vi "仪器控制2.vi"() -> ()   [LabVIEW 2012]
uses:
  <vilib>/Instr/_visa.llb/VISA Configure Serial Port (Instr).vi
panel:
  out "已循环周期数":i32
  out "电流下限":dbl
  out "电流上限":dbl
  in  "截取下限时间 2":dbl=50.0
  in  "截取上限时间 2":dbl=59.5
  in  "偏差范围下限 2":dbl=20.0
  in  "偏差范围上限 2":dbl=20.0
  in  "截取下限时间":dbl=0.75
  in  "截取上限时间":dbl=49.0
  out "当前时间值":dbl
  out "电流超出范围":bool=TRUE
  out "原始数据":dbl
  out "大小":i32
  in  "终止程序":bool
  out "x-y":u32
  out "波形图":dbl[](graph)
  out "子字符串之前 2":string
  out "双精度浮点数":dbl
  out "*(类型 *) &x":dbl
  out "实际输出电流":dbl
  out "匹配后偏移量":i32
  out "子字符串之后":string
  out "匹配子字符串":string
  out "子字符串之前":string
  out "读取缓冲区":string
  out "Serial Settings:Number of Bytes at Serial Port":u32
  out "停止按钮指示灯":bool
  out "运行按钮指示灯":bool
  in  "停止运行":bool
  in  "运行程序":bool
  in  "第一段波形持续时间(s)":dbl=49.25
  in  "循环周期数":i32=30000
  in  "0安培电流保持时长":dbl=60.0
  in  "前三段波形持续时间（s）":dbl=60.0
  in  "前两段波形持续时间（s）":dbl=59.5
  in  "Time Resolution(s)":dbl=0.03
  in  "IR":dbl=50.0
  out "第一周期近似波形图":dbl[](graph)
  # "配置"
  # "检测"
  # "Time Resolution(s)不能小于0.03否则时间将特别不准"
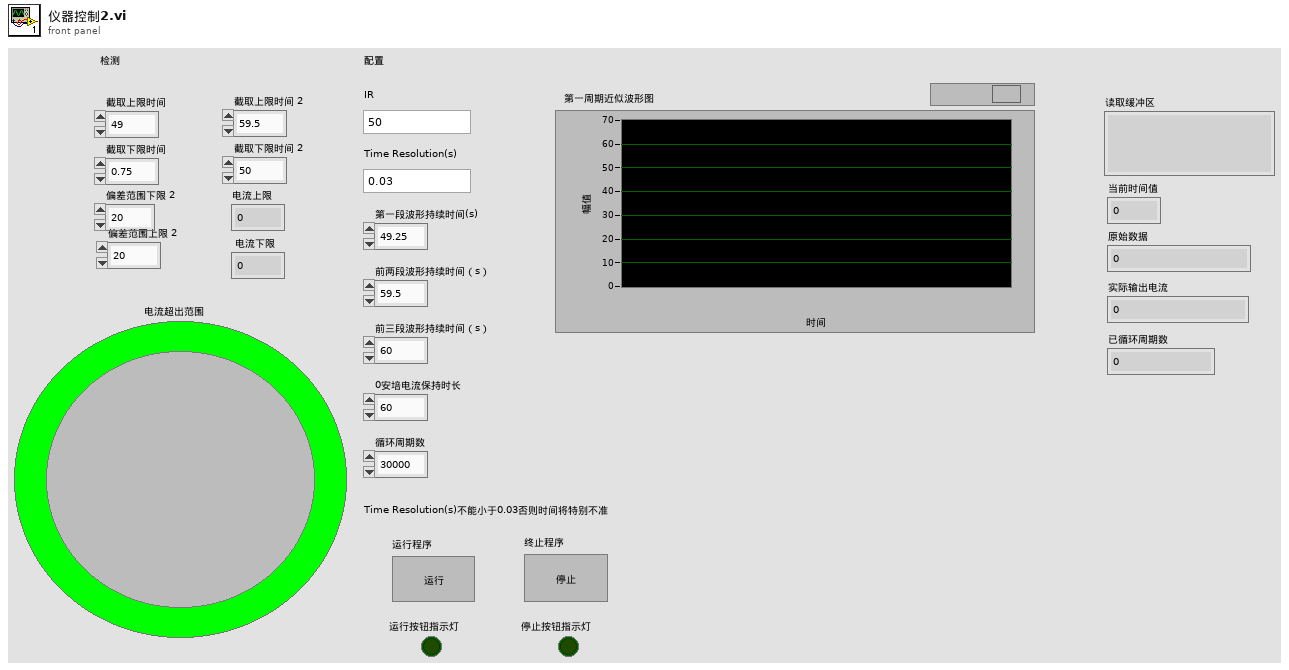
[diagram p1: front panel]
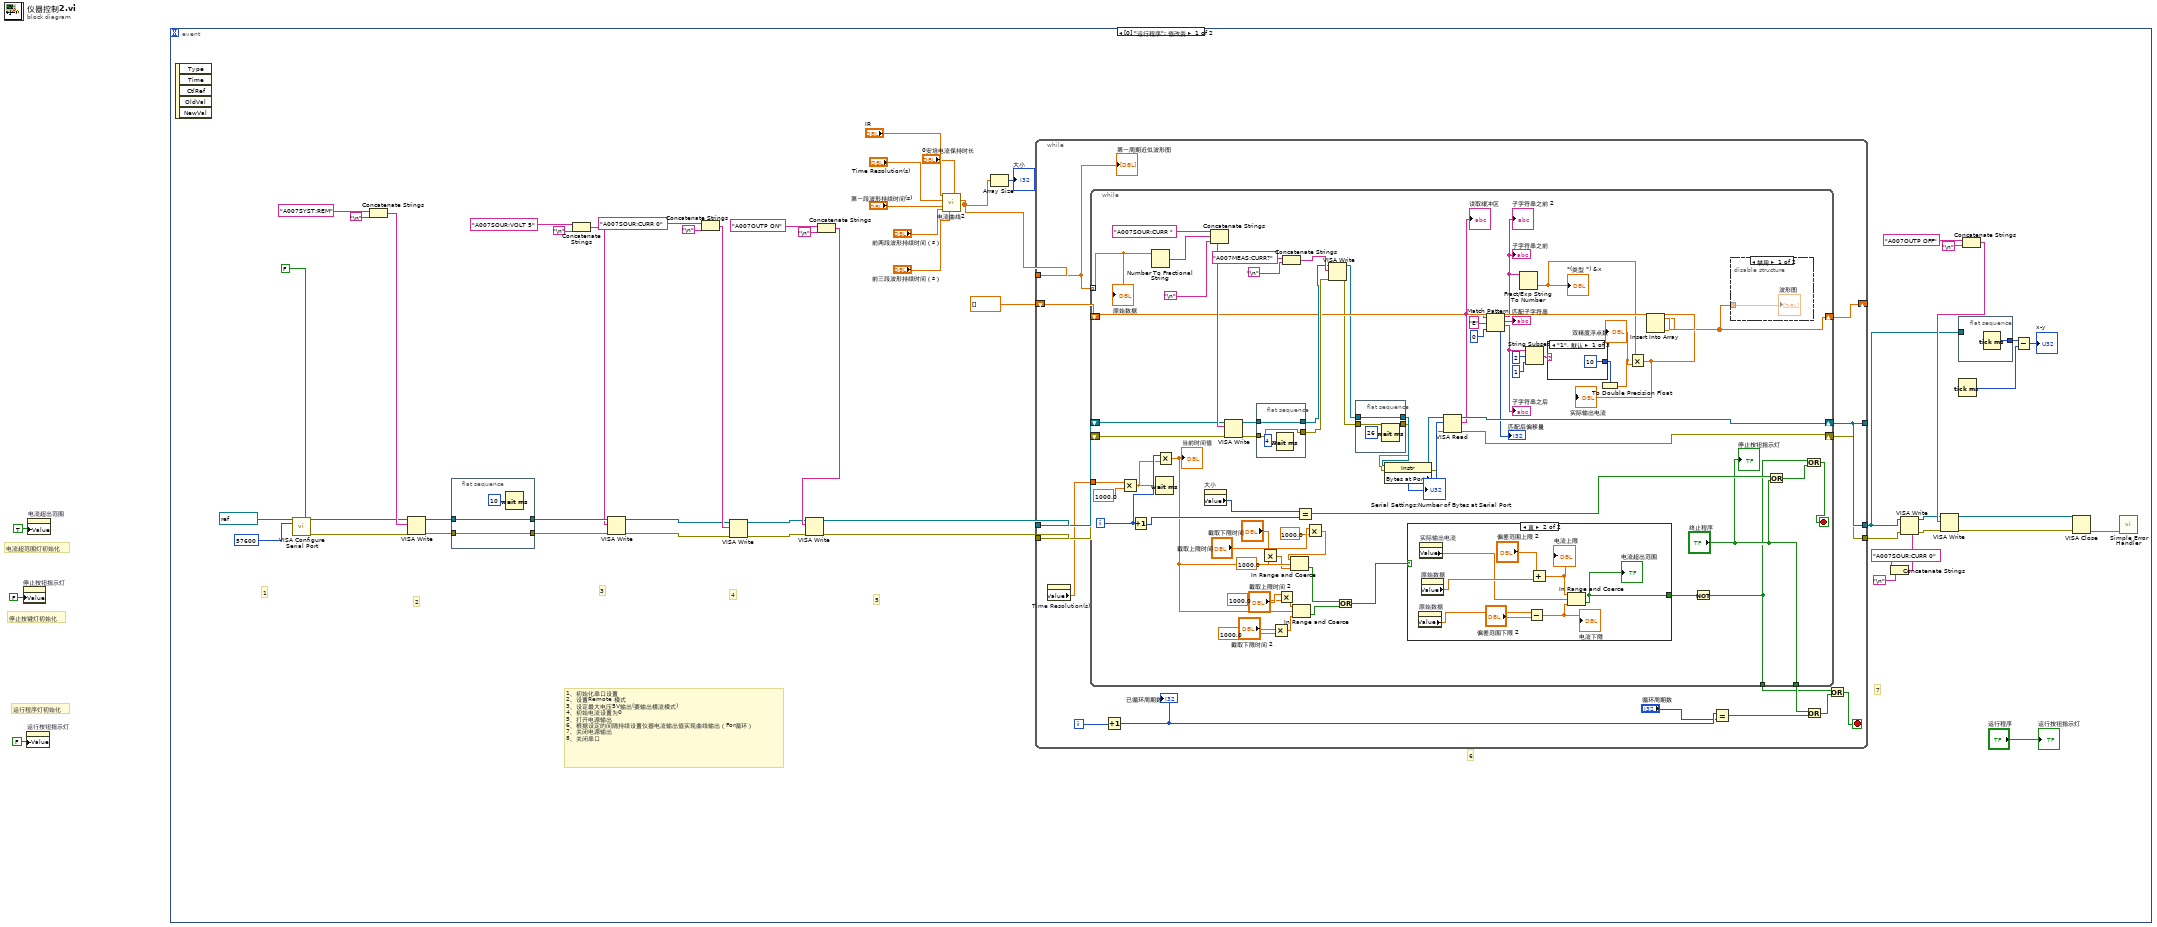
[diagram p0: block diagram]
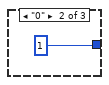
[diagram p2: hidden frame]
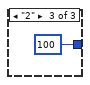
[diagram p3: hidden frame]
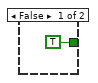
[diagram p5: hidden frame]
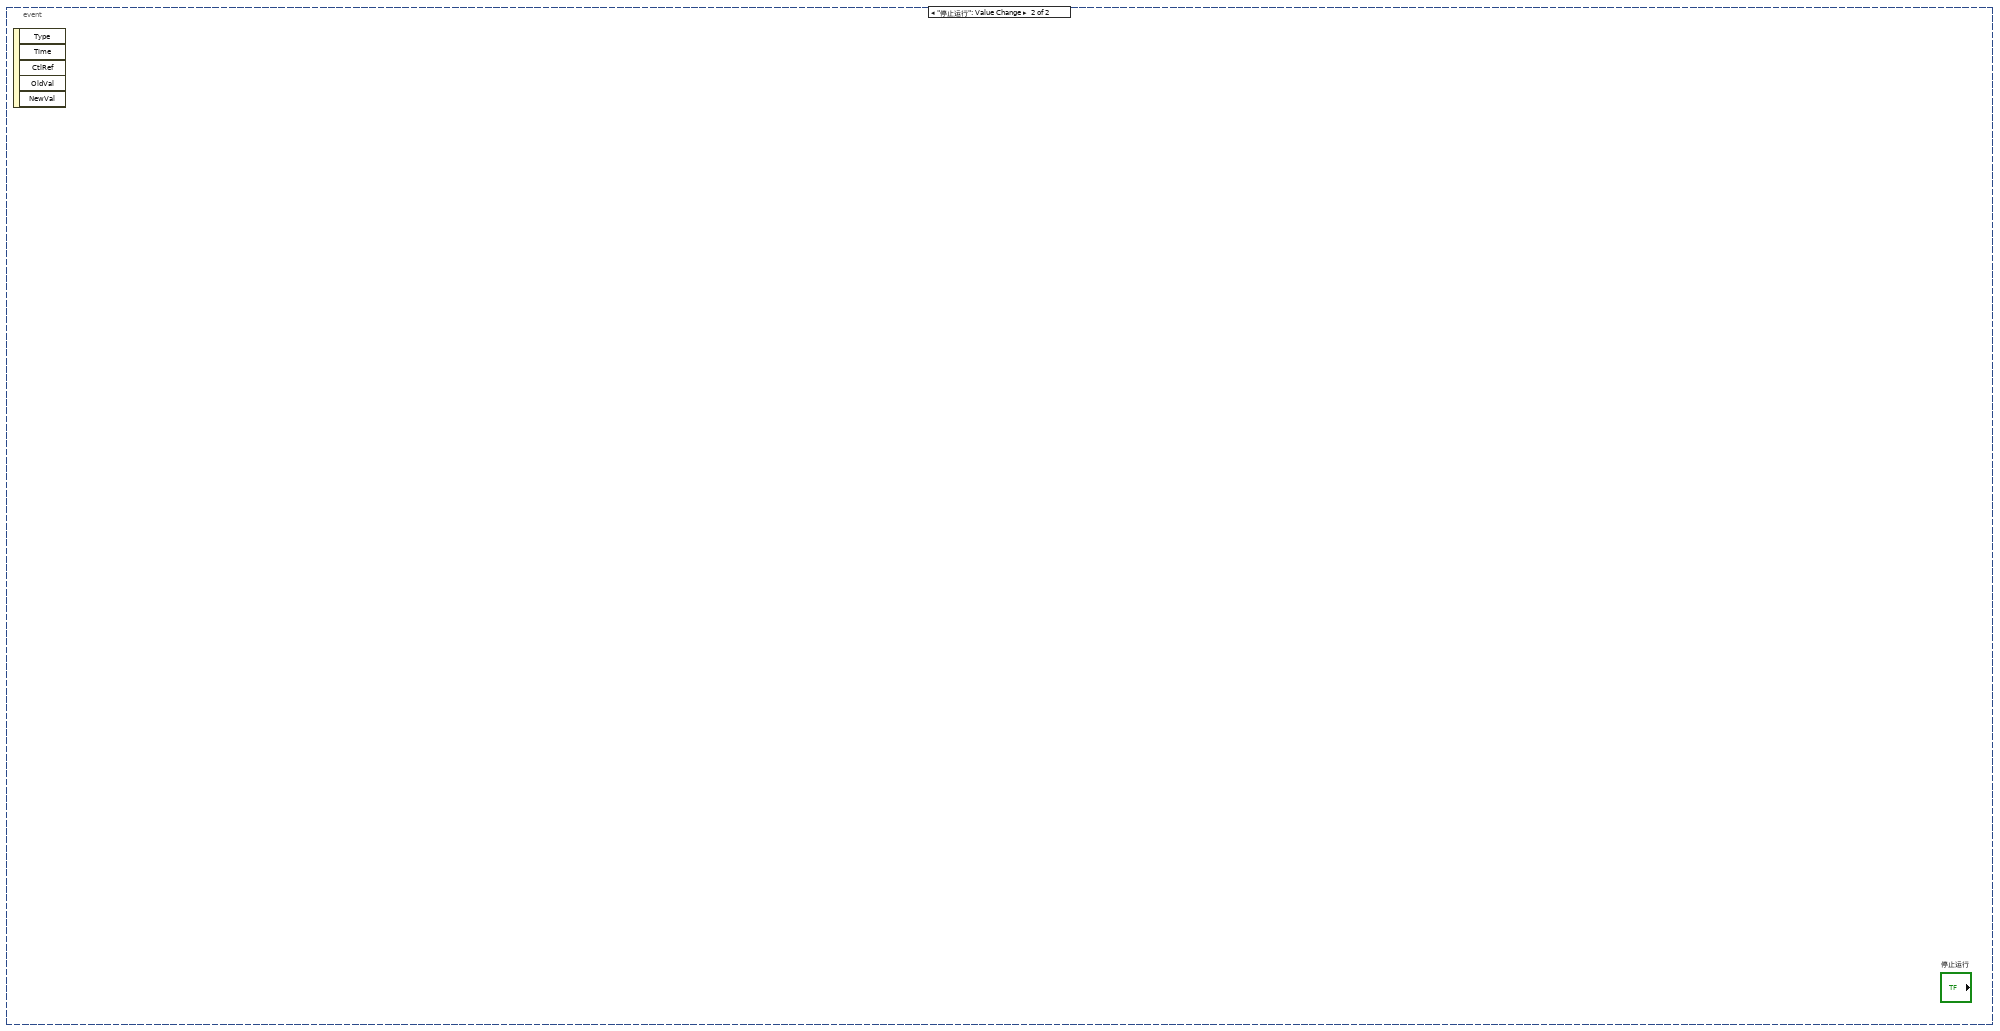
[diagram p6: hidden frame]
diagram:
  # "电流超范围灯初始化"
  # "停止按键灯初始化"
  # "运行程序灯初始化"
  n1 = property on="停止按钮指示灯" class="Bool (严格)"("Value"=FALSE ("停止按钮指示灯")) -> ()  [unwired: 2 in, 2 out]
  n2 = property on="运行按钮指示灯" class="Bool (严格)"("Value"=FALSE ("运行按钮指示灯")) -> ()  [unwired: 2 in, 2 out]
  n3 = property on="电流超出范围" class="Bool (严格)"("Value"=TRUE ("电流超出范围")) -> ()  [unwired: 2 in, 2 out]
  n4 = event shown="[0] \"运行程序\": 值改变" {
    selector: _ -> [_ _]
    dyn-events: _ -> [_ _]
    timeout: _ -> [_ _]
    event "运行程序": Value Change {
      # "6"
      # "7"
      # "5"
      # "4"
      # "3"
      # "2"
      # "1"
      # "1、初始化串口设置\n2、设置Remote 模式\n3、设定最大电压5V输出(要输出横流模式)\n4、初始电流设置为0\n5、打开电源输出\n6、根据设定的间隔持续设置仪器电流输出值实现曲线输出（For循环）\n7、关闭电源输出\n8、关闭串口"
      n5 = event-data() -> ()  [unwired: 1 in, 5 out]
      n6 = call-poly "VISA Configure Serial Port"("VISA resource name"=refnum<visa-resource-name> "COM3", "Enable Termination\nChar (T)"=FALSE ("Enable Termination\nChar (T)"), "baud rate (9600)"=u32 57600) -> ("VISA resource name out"=w48:refnum<visa-resource-name>, "error out"=w47:errorcluster)  [unwired: 11 in]
      n7 = Concatenate Strings("A007SYST:REM" ("字符串"), "\n") -> (w53:string)
      n8 = VISA Write(VISA resource name=w48, write buffer=w53, error in (no error)=w47) -> (VISA resource name out=w56:refnum<visa-resource-name>, error out=w55:errorcluster)  [unwired: 1 out]
      n9 = flat-sequence {
        tunnel: w56 -> [w161]
        tunnel: [w161] -> w45
        tunnel: w55 -> [w160]
        tunnel: [w160] -> w44
        frame #0 {
          n10 = Wait (ms)(milliseconds to wait=u32 10 ("等待时间（毫秒）")) -> ()  [unwired: 1 out]
        }
      }
      n11 = Concatenate Strings("A007SOUR:VOLT 5" ("字符串"), "\n") -> (w41:string)
      n12 = VISA Write(VISA resource name=w45, write buffer=w41, error in (no error)=w44) -> (VISA resource name out=w37:refnum<visa-resource-name>, error out=w36:errorcluster)  [unwired: 1 out]
      n13 = Concatenate Strings("A007SOUR:CURR 0" ("字符串"), "\n") -> (w40:string)
      n14 = VISA Write(VISA resource name=w37, write buffer=w40, error in (no error)=w36) -> (VISA resource name out=w32:refnum<visa-resource-name>, error out=w31:errorcluster)  [unwired: 1 out]
      n15 = Concatenate Strings("A007OUTP ON" ("字符串"), "\n") -> (w33:string)
      n16 = VISA Write(VISA resource name=w32, write buffer=w33, error in (no error)=w31) -> (VISA resource name out=w30:refnum<visa-resource-name>, error out=w29:errorcluster)  [unwired: 1 out]
      n17 = call "电流曲线2.vi"("0安培电流保持时长"="0安培电流保持时长", "总持续时间3"="前三段波形持续时间（s）", "总持续时间2"="前两段波形持续时间（s）", "总持续时间1"="第一段波形持续时间(s)", "时间分辨率"="Time Resolution(s)", "IR"="IR") -> ("最终电流值"=w12:dbl[])  [unwired: 5 in]
      n18 = Array Size(array=w12) -> (size(s)=→"大小":i32)
      n19 = while {
        tunnel: w30 -> [w72]
        tunnel: w29 -> [w71]
        tunnel: [w61] -> w7
        tunnel: [w60] -> w6
        tunnel: w12 -> [w69]
        shift-right: [w67] -> _
        shift-left: dbl[] [] ("波形图") -> [w68]
        tunnel: [w61] -> _
        i -> [w66]
        stop <- w59 stop-if-true
        n20 = property on="Time Resolution(s)" class="DigNum (严格)"() -> ("Value"=w70:dbl)  [unwired: 2 in, 2 out]
        n21 = while {
          tunnel: w69 -> [w131] mode=indexing
          tunnel: w70 -> [w133]
          shift-right: [w122] -> w60
          shift-left: w71 -> [w136]
          shift-right: [w123] -> w61
          shift-left: w72 -> [w137]
          shift-right: [w120] -> w67
          shift-left: w68 -> [w121]
          tunnel: ["终止程序"] -> w62
          tunnel: [w111] -> w57
          i -> [w113]
          stop <- w114 stop-if-true
          n22 = Multiply(x=w133, y=1000.0) -> (x*y=w112:dbl)
          n23 = Increment(x=w113) -> (x+1=w119:i32)
          n24 = Number To Fractional String(number=w131) -> (F-format string=w134:string)  [unwired: 3 in]
          n25 = Wait (ms)(milliseconds to wait=w112) -> ()  [unwired: 1 out]
          n26 = Multiply(x=w113, y=w112) -> (x*y=w110:dbl)
          "当前时间值" <- w110
          n27 = property on="大小" class="DigNum (严格)"() -> ("Value"=w118:i32)  [unwired: 2 in, 2 out]
          n28 = Concatenate Strings("A007SOUR:CURR " ("字符串"), w134, "\n") -> (w138:string)
          n29 = VISA Write(VISA resource name=w137, write buffer=w138, error in (no error)=w136) -> (VISA resource name out=w127:refnum<visa-resource-name>, error out=w126:errorcluster)  [unwired: 1 out]
          n30 = flat-sequence {
            tunnel: w127 -> [w157]
            tunnel: w126 -> [w156]
            tunnel: [w157] -> w124
            tunnel: [w156] -> w125
            frame #0 {
              n31 = Wait (ms)(milliseconds to wait=u32 4 ("等待时间（毫秒）")) -> ()  [unwired: 1 out]
            }
          }
          n32 = Multiply(x="截取下限时间", y=1000.0) -> (x*y=w104:dbl)
          n33 = Multiply(x="截取下限时间 2", y=1000.0) -> (x*y=w98:dbl)
          n34 = Multiply(x="截取上限时间 2", y=1000.0) -> (x*y=w95:dbl)
          n35 = Concatenate Strings("A007MEAS:CURR?" ("字符串"), "\n") -> (w130:string)
          n36 = In Range and Coerce(upper limit=w95, x=w110, lower limit=w98) -> (In Range?=w103:bool)  [unwired: 1 out]
          n37 = Equal?(x=w118, y=w119) -> (x = y?=w117:bool)
          n38 = Multiply(x="截取上限时间", y=1000.0) -> (x*y=w107:dbl)
          n39 = In Range and Coerce(upper limit=w107, x=w110, lower limit=w104) -> (In Range?=w102:bool)  [unwired: 1 out]
          n40 = VISA Write(VISA resource name=w124, write buffer=w130, error in (no error)=w125) -> (VISA resource name out=w90:refnum<visa-resource-name>, error out=w89:errorcluster)  [unwired: 1 out]
          n41 = Or(x=w102, y=w103) -> (x .or. y?=w101:bool)
          n42 = flat-sequence {
            tunnel: w90 -> [w144]
            tunnel: [w144] -> w88
            tunnel: w89 -> [w143]
            tunnel: [w143] -> w87
            frame #0 {
              n43 = Wait (ms)(milliseconds to wait=u32 26 ("等待时间（毫秒）")) -> ()  [unwired: 1 out]
            }
          }
          n44 = property class="Instr"(reference=w88, error in=w87) -> (reference out=w85:refnum<visa-resource-name>, error out=w84:errorcluster, "Bytes at Port"=w86:u32)
          "Serial Settings:Number of Bytes at Serial Port" <- w86
          n45 = case shown="真" w101 {
            tunnel: [TRUE w148] -> w94
            frame False {
            }
            frame True {
              n46 = property on="原始数据" class="DigNum (严格)"() -> ("Value"=w151:dbl)  [unwired: 2 in, 2 out]
              n47 = property on="实际输出电流" class="DigNum (严格)"() -> ("Value"=w149:dbl)  [unwired: 2 in, 2 out]
              n48 = property on="原始数据" class="DigNum (严格)"() -> ("Value"=w152:dbl)  [unwired: 2 in, 2 out]
              n49 = Subtract(x=w151, y="偏差范围下限 2") -> (x-y=w153:dbl)
              "电流下限" <- w153
              n50 = Add(x="偏差范围上限 2", y=w152) -> (x+y=w155:dbl)
              "电流上限" <- w155
              n51 = In Range and Coerce(upper limit=w155, x=w149, lower limit=w153) -> (In Range?=w148:bool)  [unwired: 1 out]
              "电流超出范围" <- w148
            }
          }
          n52 = VISA Read(VISA resource name=w85, byte count=w86, error in (no error)=w84) -> (VISA resource name out=w123:refnum<visa-resource-name>, read buffer=w83:string, error out=w122:errorcluster)  [unwired: 1 out]
          "读取缓冲区" <- w83
          n53 = Match Pattern(string=w83, regular expression="E" ("正则表达式"), offset (0)=0 ("偏移量(0)")) -> (before substring=w73:string, match substring=→"匹配子字符串":string, after substring=w78:string, offset past match=→"匹配后偏移量":i32)
          "子字符串之前" <- w73
          "子字符串之后" <- w78
          "子字符串之前 2" <- w73
          n54 = Fract/Exp String To Number(string=w73) -> (number=w91:dbl)  [unwired: 3 in, 1 out]
          "*(类型 *) &x" <- w91
          n55 = String Subset(string=w78, offset (0)=2 ("偏移量(0)"), length (rest)=1 ("长度（剩余）")) -> (substring=w75:string)
          n56 = case shown="\"1\", 默认" w75 {
            tunnel: [10 1 100] -> w74
            frame "1", Default {
            }
            frame "0" {
            }
            frame "2" {
            }
          }
          n57 = To Double Precision Float(number=w74) -> (double precision float=w92:dbl)
          "双精度浮点数" <- w92
          n58 = Multiply(x=w91, y=w92) -> (x*y=w93:dbl)
          "实际输出电流" <- w93
          n59 = Insert Into Array(array=w121, new element=w93) -> (w120:dbl[])  [unwired: 1 in]
          n60 = Not(x=w94) -> (.not. x?=w111:bool)
          n61 = disable-structure shown="禁用" {
            disable-tunnel: w120 -> [w146 _]
            frame Disabled {
              "波形图" <- w146
            }
            frame Enabled {
            }
          }
          n62 = Or(x=w117, y="终止程序") -> (x .or. y?=w115:bool)
          n63 = Or(x=w111, y=w115) -> (x .or. y?=w114:bool)
          "停止按钮指示灯" <- "终止程序"
          "原始数据" <- w131
        }
        n64 = Increment(x=w66) -> (x+1=w65:i32)
        "已循环周期数" <- w65
        n65 = Equal?(x=w65, y="循环周期数") -> (x = y?=w63:bool)
        n66 = Or(x=w62, y=w63) -> (x .or. y?=w58:bool)
        n67 = Or(x=w57, y=w58) -> (x .or. y?=w59:bool)
        "第一周期近似波形图" <- w69
      }
      n68 = Concatenate Strings("A007SOUR:CURR 0", "\n") -> (w10:string)
      n69 = VISA Write(VISA resource name=w7, write buffer=w10, error in (no error)=w6) -> (VISA resource name out=w5:refnum<visa-resource-name>, error out=w4:errorcluster)  [unwired: 1 out]
      n70 = flat-sequence {
        tunnel: w7 -> [_]
        tunnel: [w159] -> w15
        frame #0 {
          n71 = Tick Count (ms)() -> (millisecond timer value=w159:u32)
        }
      }
      n72 = Tick Count (ms)() -> (millisecond timer value=w14:u32)
      n73 = Concatenate Strings("A007OUTP OFF" ("字符串"), "\n") -> (w28:string)
      n74 = VISA Write(VISA resource name=w5, write buffer=w28, error in (no error)=w4) -> (VISA resource name out=w26:refnum<visa-resource-name>, error out=w25:errorcluster)  [unwired: 1 out]
      n75 = Subtract(x=w15, y=w14) -> (x-y=→"x-y":u32)
      n76 = VISA Close(VISA resource name=w26, error in (no error)=w25) -> (error out=w51:errorcluster)
      n77 = call <vilib>:"Simple Error Handler.vi"("error in (no error)"=w51) -> ()  [unwired: 4 in, 5 out]
      "运行按钮指示灯" <- "运行程序"
    }
    event "停止运行": Value Change {
      n78 = event-data() -> ()  [unwired: 1 in, 5 out]
    }
  }
